vi "Begin.vi"(8 "error in":errorcluster) -> (0 "error out":errorcluster)   [LabVIEW 2016]
doc: "Called before other user functions, this VI is expected to open initial I/O refnums, load in file data, and do all program initialization. Notice that the <B>error out</B> terminal is simply used for data flow. Wiring it to other structures or subVIs ensures that this VI runs first."
uses:
  <vilib>/Rock Robotics/WPI/DriverStation/WPI_DriverStationRobotMode2.ctl
  <vilib>/Rock Robotics/WPI/Joystick/WPI_JoystickDeviceEnum.ctl
  <vilib>/Rock Robotics/WPI/ThirdParty/CanMotor/TalonSRX/WPI_CANTalonSRX_APIFeedbackSelect.ctl
  <vilib>/Rock Robotics/WPI/Solenoid/WPI_SolenoidChannel.ctl
  <vilib>/Rock Robotics/SystemInterfaces/spilib/spi_bus.ctl
  <vilib>/Rock Robotics/SystemInterfaces/DIO/FPGA_DIOPWMChannel.ctl
  <vilib>/Rock Robotics/SystemInterfaces/AI/FPGA_AIChannel.ctl
  <vilib>/Rock Robotics/WPI/ThirdParty/CanMotor/TalonSRX/WPI_CANTalonSRX_BrakeOverride.ctl
  Robot Global Data.vi
  <vilib>/Rock Robotics/Network Tables/NT Write String Array.vi
  <vilib>/Rock Robotics/WPI/Solenoid/WPI_SolenoidOpenDouble.vi
  <vilib>/Rock Robotics/WPI/Gyro/WPI_GyroXRS450_SPI_Open.vi
  <vilib>/Rock Robotics/WPI/MotorControl/WPI_MotorControlOpen VictorSP.vi
  Systems/Global 1.vi
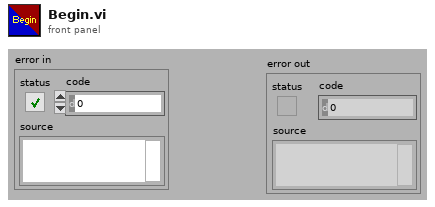
[diagram p1: front panel]
types:
  T1 = typedef "WPI_SolenoidChannel.ctl" = enum8{"Solenoid 0", "Solenoid 1", "Solenoid 2", "Solenoid 3", "Solenoid 4", "Solenoid 5", "Solenoid 6", "Solenoid 7", "Invalid"}
  T2 = typedef "WPI_CANTalonSRX_BrakeOverride.ctl" = enum8{"No Override", "Override to Coast", "Override to Brake"}
  T3 = typedef "FPGA_DIOPWMChannel.ctl" = enum8{"PWM 0", "PWM 1", "PWM 2", "PWM 3", "PWM 4", "PWM 5", "PWM 6", "PWM 7", "PWM 8", "PWM 9", "PWM MXP 0", "PWM MXP 1", "PWM MXP 2", "PWM MXP 3", "PWM MXP 4", "PWM MXP 5", "PWM MXP 6", "PWM MXP 7", "PWM MXP 8", "PWM MXP 9", "Invalid"}
  T4 = typedef "FPGA_AIChannel.ctl" = enum8{"AI 0", "AI 1", "AI 2", "AI 3", "AI MXP 0", "AI MXP 1", "AI MXP 2", "AI MXP 3", "Invalid"}
  T5 = typedef "spi_bus.ctl" = enum16{"SPI On-Board, CS0", "SPI On-Board, CS1", "SPI On-Board, CS2", "SPI On-Board, CS3", "SPI MXP", "Invalid"}
  T6 = typedef "WPI_CANTalonSRX_APIFeedbackSelect.ctl" = enum16{"Digital Quadrature Encoder", "Analog Potentiometer", "Analog Encoder", "Count on Quad-A (Rising-Edge)", "Count on Quad-A (Falling-Edge)", "CTR Magnetic Enc (Absolute)", "CTR Magnetic Enc (Relative)", "Pulse Width"}
  T7 = typedef "WPI_JoystickDeviceEnum.ctl" = enum16{"USB 0", "USB 1", "USB 2", "USB 3", "USB 4", "USB 5"}
  T8 = typedef "WPI_DriverStationRobotMode2.ctl" = enum16{"Autonomous Disabled", "Autonomous Enabled", "Teleop Disabled", "Teleop Enabled", "Disconnected", "Finish", "Test Disabled", "Test Enabled", "Emergency Stopped"}
  T9 = typedef "WPI_MotorControlDeviceRef.ctl" = cluster{"DeviceStatus":errorcluster, "Type":T10, "PWM":cluster{"PWM Channel":T3, "DeadBand":T11}, "CAN":cluster{"Device Number":u8, "SetOutput VI Ref":variant, "GetOutput VI Ref":variant, "Enable VI Ref":variant, "Disable VI Ref":variant, "Data":variant}, "Invert":bool}
  T10 = typedef "WPI_MotorControlType.ctl" = enum16{"PWM", "CAN"}
  T11 = typedef "WPI_PWMDeadband.ctl" = cluster{"Name":string, "maxPositivePwm":i32, "minPositivePwm":i32, "centerPwm":i32, "maxNegativePwm":i32, "minNegativePwm":i32, "angularRange":u16}
  T12 = typedef "WPI_JoystickDevRef.ctl" = cluster{"Device":T7}
  T13 = typedef "WPI_SolenoidDevRef.ctl" = cluster{"DevStatus":errorcluster, "Pneumatics Control Module":u8, "Forward Solenoid Channel":T1, "Reverse Solenoid Channel":T1}
  T14 = typedef "WPI_ServoDeviceRef.ctl" = cluster{"DeviceStatus":errorcluster, "PWM Channel":T3, "DeadBand":T11}
  T15 = typedef "WPI_AnalogChannelDevRef.ctl" = cluster{"DevStatus":errorcluster, "Analog Channel":T4}
  T16 = typedef "WPI_GyroDevRef.ctl" = cluster{"DevStatus":errorcluster, "Analog Channel":T4, "Offset":dbl, "Gain (VoltsPerDegree/Second)":dbl, "Gyro Type":enum16{"Analog", "XRS450"}, "Handle":i32, "SPI Bus":T5, "Device Found":bool, "Sample Rate":dbl, "Calibrate On Open":bool}
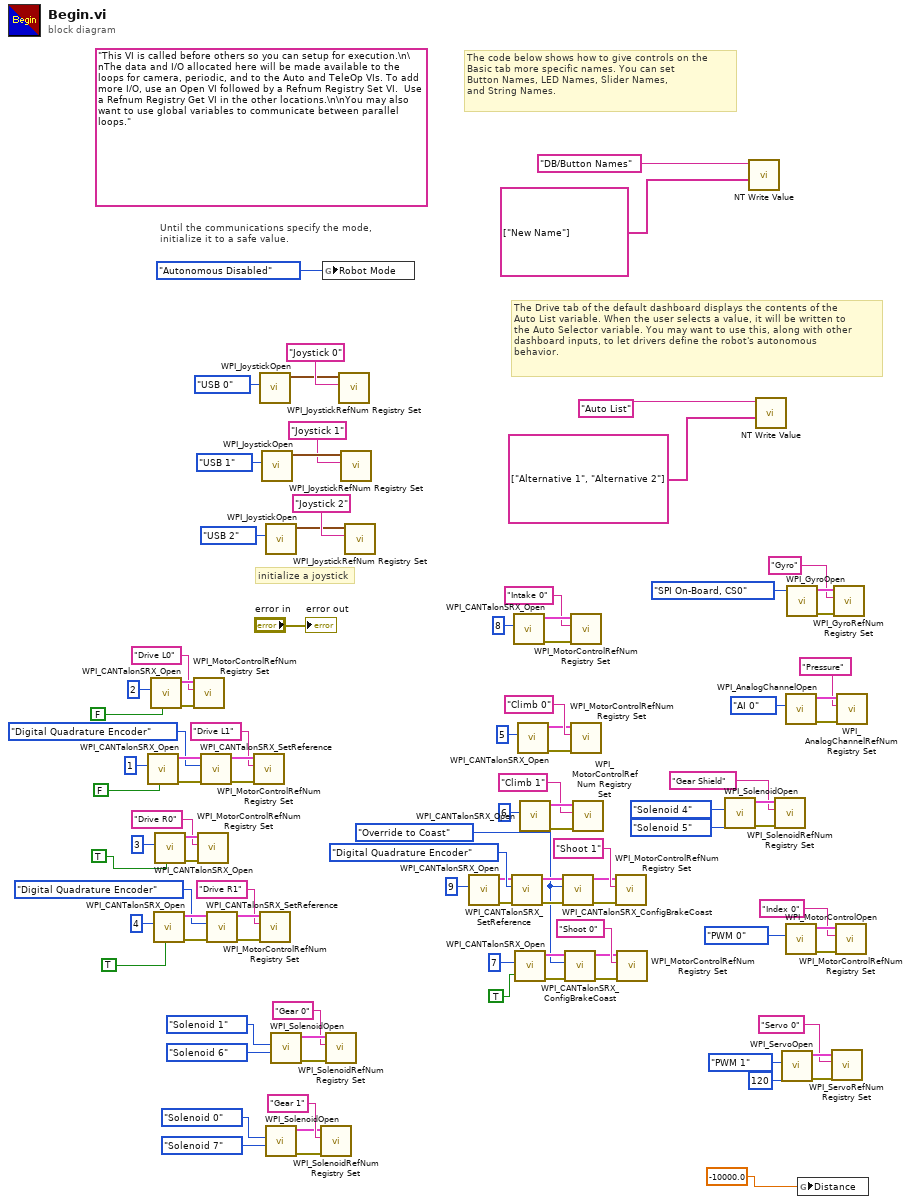
[diagram p0: block diagram]
diagram:
  w8 = WPI_CANTalonSRX_BrakeOverride."Override to Coast" ("Brake / Coast Mode")
  (unwired) "This VI is called before others so you can setup for execution.\n\nThe data and I/O allocated here will be made available to the loops for camera, periodic, and to the Auto and TeleOp VIs. To add more I/O, use an Open VI followed by a Refnum Registry Set VI.  Use a Refnum Registry Get VI in the other locations.\n\nYou may also want to use global variables to communicate between parallel loops."
  # "The Drive tab of the default dashboard displays the contents of the\nAuto List variable. When the user selects a value, it will be written to\nthe Auto Selector variable. You may want to use this, along with other\ndashboard inputs, to let drivers define the robot's autonomous\nbehavior."
  # "The code below shows how to give controls on the\nBasic tab more specific names. You can set\nButton Names, LED Names, Slider Names,\nand String Names."
  # "initialize a joystick"
  # "Until the communications specify the mode,\ninitialize it to a safe value."
  n1 = call <vilib>:"WPI_CANTalonSRX_Open.vi"("Invert"=FALSE, "Device Number"=u8 1) -> ("error out"=w85:errorcluster, "CAN Talon SRX Ref"=w86:T9)  [unwired: 8 in]
  n2 = call <vilib>:"WPI_CANTalonSRX_Open.vi"("Invert"=FALSE, "Device Number"=u8 2) -> ("error out"=w79:errorcluster, "CAN Talon SRX Ref"=w80:T9)  [unwired: 8 in]
  n3 = call <vilib>:"WPI_CANTalonSRX_Open.vi"("Invert"=TRUE, "Device Number"=u8 4) -> ("error out"=w84:errorcluster, "CAN Talon SRX Ref"=w83:T9)  [unwired: 8 in]
  n4 = call <vilib>:"WPI_CANTalonSRX_Open.vi"("Invert"=TRUE, "Device Number"=u8 3) -> ("error out"=w76:errorcluster, "CAN Talon SRX Ref"=w77:T9)  [unwired: 8 in]
  n5 = call <vilib>:"WPI_MotorControlRefNum Registry Set.vi"("error in (no error)"=w79, "refnum name"="Drive L0", "MotorControlDevRef"=w80) -> ()  [unwired: 7 in, 2 out]
  n6 = call <vilib>:"WPI_MotorControlRefNum Registry Set.vi"("error in (no error)"=w76, "refnum name"="Drive R0", "MotorControlDevRef"=w77) -> ()  [unwired: 7 in, 2 out]
  n7 = call <vilib>:"WPI_CANTalonSRX_SetReference.vi"("error in (no error)"=w85, "Feedback Reference"=WPI_CANTalonSRX_APIFeedbackSelect."Digital Quadrature Encoder", "CAN Talon SRX Ref"=w86) -> ("error out"=w87:errorcluster, "CAN Talon SRX Ref"=w88:T9)  [unwired: 7 in]
  n8 = call <vilib>:"WPI_CANTalonSRX_SetReference.vi"("error in (no error)"=w84, "Feedback Reference"=WPI_CANTalonSRX_APIFeedbackSelect."Digital Quadrature Encoder", "CAN Talon SRX Ref"=w83) -> ("error out"=w82:errorcluster, "CAN Talon SRX Ref"=w81:T9)  [unwired: 7 in]
  n9 = call <vilib>:"WPI_MotorControlRefNum Registry Set.vi"("error in (no error)"=w87, "refnum name"="Drive L1", "MotorControlDevRef"=w88) -> ()  [unwired: 7 in, 2 out]
  n10 = call <vilib>:"WPI_JoystickOpen.vi"("JoystickDevice"=WPI_JoystickDeviceEnum."USB 0") -> ("JoystickDevRef"=w101:T12)  [unwired: 10 in]
  n11 = call <vilib>:"WPI_MotorControlRefNum Registry Set.vi"("error in (no error)"=w82, "refnum name"="Drive R1", "MotorControlDevRef"=w81) -> ()  [unwired: 7 in, 2 out]
  n12 = call <vilib>:"WPI_JoystickOpen.vi"("JoystickDevice"=WPI_JoystickDeviceEnum."USB 1") -> ("JoystickDevRef"=w93:T12)  [unwired: 10 in]
  n13 = call <vilib>:"WPI_JoystickOpen.vi"("JoystickDevice"=WPI_JoystickDeviceEnum."USB 2") -> ("JoystickDevRef"=w90:T12)  [unwired: 10 in]
  n14 = call-poly <vilib>:"WPI_SolenoidOpen.vi"("Reverse Solenoid Channel"=WPI_SolenoidChannel."Solenoid 7", "Forward Solenoid Channel"=WPI_SolenoidChannel."Solenoid 0") -> ("error out"=w61:errorcluster, "SolenoidDevRef"=w62:T13)  [unwired: 8 in]
  n15 = call-poly <vilib>:"WPI_SolenoidOpen.vi"("Reverse Solenoid Channel"=WPI_SolenoidChannel."Solenoid 6", "Forward Solenoid Channel"=WPI_SolenoidChannel."Solenoid 1") -> ("error out"=w66:errorcluster, "SolenoidDevRef"=w65:T13)  [unwired: 8 in]
  n16 = call <vilib>:"WPI_SolenoidRefNum Registry Set.vi"("error in (no error)"=w61, "refnum name"="Gear 1", "SolenoidDevRef"=w62) -> ()  [unwired: 7 in, 2 out]
  n17 = global write "Robot Global Data.vi" "Robot Mode"(WPI_DriverStationRobotMode2."Autonomous Disabled" ("Robot Mode")) -> ()
  n18 = call <vilib>:"WPI_SolenoidRefNum Registry Set.vi"("error in (no error)"=w66, "refnum name"="Gear 0", "SolenoidDevRef"=w65) -> ()  [unwired: 7 in, 2 out]
  n19 = call <vilib>:"WPI_JoystickRefNum Registry Set.vi"("refnum name"="Joystick 0", "JoystickDevRef"=w101) -> ()  [unwired: 8 in, 2 out]
  n20 = call <vilib>:"WPI_JoystickRefNum Registry Set.vi"("refnum name"="Joystick 1", "JoystickDevRef"=w93) -> ()  [unwired: 8 in, 2 out]
  n21 = call <vilib>:"WPI_JoystickRefNum Registry Set.vi"("refnum name"="Joystick 2", "JoystickDevRef"=w90) -> ()  [unwired: 8 in, 2 out]
  n22 = call <vilib>:"WPI_CANTalonSRX_Open.vi"("Device Number"=u8 9) -> ("error out"=w54:errorcluster, "CAN Talon SRX Ref"=w55:T9)  [unwired: 9 in]
  n23 = call <vilib>:"WPI_CANTalonSRX_SetReference.vi"("error in (no error)"=w54, "Feedback Reference"=WPI_CANTalonSRX_APIFeedbackSelect."Digital Quadrature Encoder", "CAN Talon SRX Ref"=w55) -> ("error out"=w13:errorcluster, "CAN Talon SRX Ref"=w14:T9)  [unwired: 7 in]
  n24 = call <vilib>:"WPI_CANTalonSRX_Open.vi"("Device Number"=u8 8) -> ("error out"=w69:errorcluster, "CAN Talon SRX Ref"=w70:T9)  [unwired: 9 in]
  n25 = call <vilib>:"WPI_CANTalonSRX_Open.vi"("Invert"=TRUE, "Device Number"=u8 7) -> ("error out"=w15:errorcluster, "CAN Talon SRX Ref"=w16:T9)  [unwired: 8 in]
  n26 = call <vilib>:"WPI_CANTalonSRX_Open.vi"("Device Number"=u8 5) -> ("error out"=w43:errorcluster, "CAN Talon SRX Ref"=w42:T9)  [unwired: 9 in]
  n27 = call <vilib>:"WPI_CANTalonSRX_Open.vi"("Device Number"=u8 6) -> ("error out"=w40:errorcluster, "CAN Talon SRX Ref"=w41:T9)  [unwired: 9 in]
  n28 = call <vilib>:"WPI_CANTalonSRX_ConfigBrakeCoast.vi"("error in (no error)"=w13, "Brake / Coast Mode"=w8, "CAN Talon SRX Ref"=w14) -> ("error out"=w9:errorcluster, "CAN Talon SRX Ref"=w10:T9)  [unwired: 7 in]
  n29 = call <vilib>:"WPI_CANTalonSRX_ConfigBrakeCoast.vi"("error in (no error)"=w15, "Brake / Coast Mode"=w8, "CAN Talon SRX Ref"=w16) -> ("error out"=w11:errorcluster, "CAN Talon SRX Ref"=w12:T9)  [unwired: 7 in]
  n30 = call <vilib>:"WPI_MotorControlRefNum Registry Set.vi"("error in (no error)"=w69, "refnum name"="Intake 0", "MotorControlDevRef"=w70) -> ()  [unwired: 7 in, 2 out]
  n31 = call <vilib>:"WPI_MotorControlRefNum Registry Set.vi"("error in (no error)"=w43, "refnum name"="Climb 0", "MotorControlDevRef"=w42) -> ()  [unwired: 7 in, 2 out]
  n32 = call <vilib>:"WPI_MotorControlRefNum Registry Set.vi"("error in (no error)"=w40, "refnum name"="Climb 1", "MotorControlDevRef"=w41) -> ()  [unwired: 7 in, 2 out]
  n33 = call <vilib>:"WPI_MotorControlRefNum Registry Set.vi"("error in (no error)"=w9, "refnum name"="Shoot 1", "MotorControlDevRef"=w10) -> ()  [unwired: 7 in, 2 out]
  n34 = call <vilib>:"WPI_MotorControlRefNum Registry Set.vi"("error in (no error)"=w11, "refnum name"="Shoot 0", "MotorControlDevRef"=w12) -> ()  [unwired: 7 in, 2 out]
  n35 = call-poly <vilib>:"WPI_SolenoidOpen.vi"("Reverse Solenoid Channel"=WPI_SolenoidChannel."Solenoid 5", "Forward Solenoid Channel"=WPI_SolenoidChannel."Solenoid 4") -> ("error out"=w5:errorcluster, "SolenoidDevRef"=w4:T13)  [unwired: 8 in]
  n36 = call-poly <vilib>:"NT Write Value.vi"("String Array"=string[] ["New Name"], "Name"="DB/Button Names") -> ()  [unwired: 9 in, 1 out]
  n37 = call-poly <vilib>:"NT Write Value.vi"("String Array"=string[] ["Alternative 1", "Alternative 2"], "Name"="Auto List") -> ()  [unwired: 9 in, 1 out]
  n38 = call <vilib>:"WPI_SolenoidRefNum Registry Set.vi"("error in (no error)"=w5, "refnum name"="Gear Shield", "SolenoidDevRef"=w4) -> ()  [unwired: 7 in, 2 out]
  n39 = call <vilib>:"WPI_ServoOpen.vi"("Angular Range"=u16 120, "PWM Channel"=FPGA_DIOPWMChannel."PWM 1") -> ("error out"=w22:errorcluster, "ServoDeviceRef"=w21:T14)  [unwired: 8 in]
  n40 = call <vilib>:"WPI_AnalogChannelOpen.vi"("Analog Channel"=FPGA_AIChannel."AI 0") -> ("error out"=w32:errorcluster, "AIDeviceRef"=w31:T15)  [unwired: 9 in]
  n41 = call-poly <vilib>:"WPI_MotorControlOpen.vi"("PWM Channel"=FPGA_DIOPWMChannel."PWM 0") -> ("error out"=w36:errorcluster, "MotorControlDeviceRef"=w35:T9)  [unwired: 9 in]
  n42 = call-poly <vilib>:"WPI_GyroOpen.vi"("SPI Bus"=spi_bus."SPI On-Board, CS0") -> ("error out"=w49:errorcluster, "GyroDevRef"=w48:T16)  [unwired: 9 in]
  n43 = global write "Global 1.vi" "Distance"(-10000.0) -> ()
  n44 = call <vilib>:"WPI_ServoRefNum Registry Set.vi"("error in (no error)"=w22, "refnum name"="Servo 0", "ServoDeviceRef"=w21) -> ()  [unwired: 7 in, 2 out]
  n45 = call <vilib>:"WPI_GyroRefNum Registry Set.vi"("error in (no error)"=w49, "refnum name"="Gyro", "GyroDevRef"=w48) -> ()  [unwired: 7 in, 2 out]
  n46 = call <vilib>:"WPI_MotorControlRefNum Registry Set.vi"("error in (no error)"=w36, "refnum name"="Index 0", "MotorControlDevRef"=w35) -> ()  [unwired: 7 in, 2 out]
  n47 = call <vilib>:"WPI_AnalogChannelRefNum Registry Set.vi"("error in (no error)"=w32, "refnum name"="Pressure", "AIDeviceRef"=w31) -> ()  [unwired: 7 in, 2 out]
  "error out" <- "error in"
